vi "LV_vs_PY_timing.vi"() -> ()   [LabVIEW 2021]
panel:
  in  "Fiducials array":path=path "C:/Users/sindh/Desktop/LabVIEW with Python/fiducials.txt"
  out "LV time":dbl
  out "Gantry Fiducials":dbl[](array[numeric])=[574.866049, -722.708823, -78.709075, 574.794272, -905.497716, -78.957629, 575.365932, -722.708925, -78.709081, 575.294318, -905.497893, -78.957622]
  out "XYZTheta":dbl[](array[numeric])
  out "PY time":dbl
  out "XYZTheta 2":dbl[](array[numeric])
  in  "Run LV":bool
  in  "Python version":string="3.6"
  in  "python function name":string="find_component_center"
  in  "python module path":path=path "C:/Users/sindh/Desktop/LabVIEW with Python/test_python.py"
  in  "Run PY":bool
  out "error out":errorcluster
  in  "error in (no error)":errorcluster
  in  "stop":bool
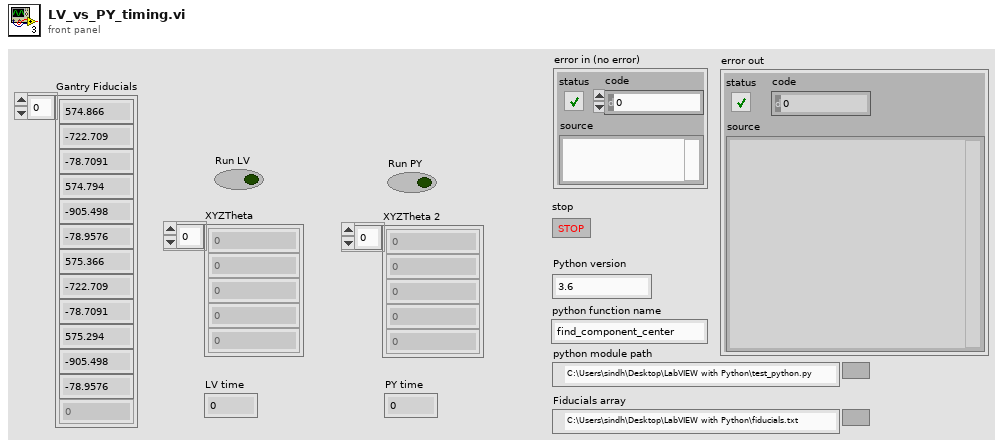
[diagram p1: front panel]
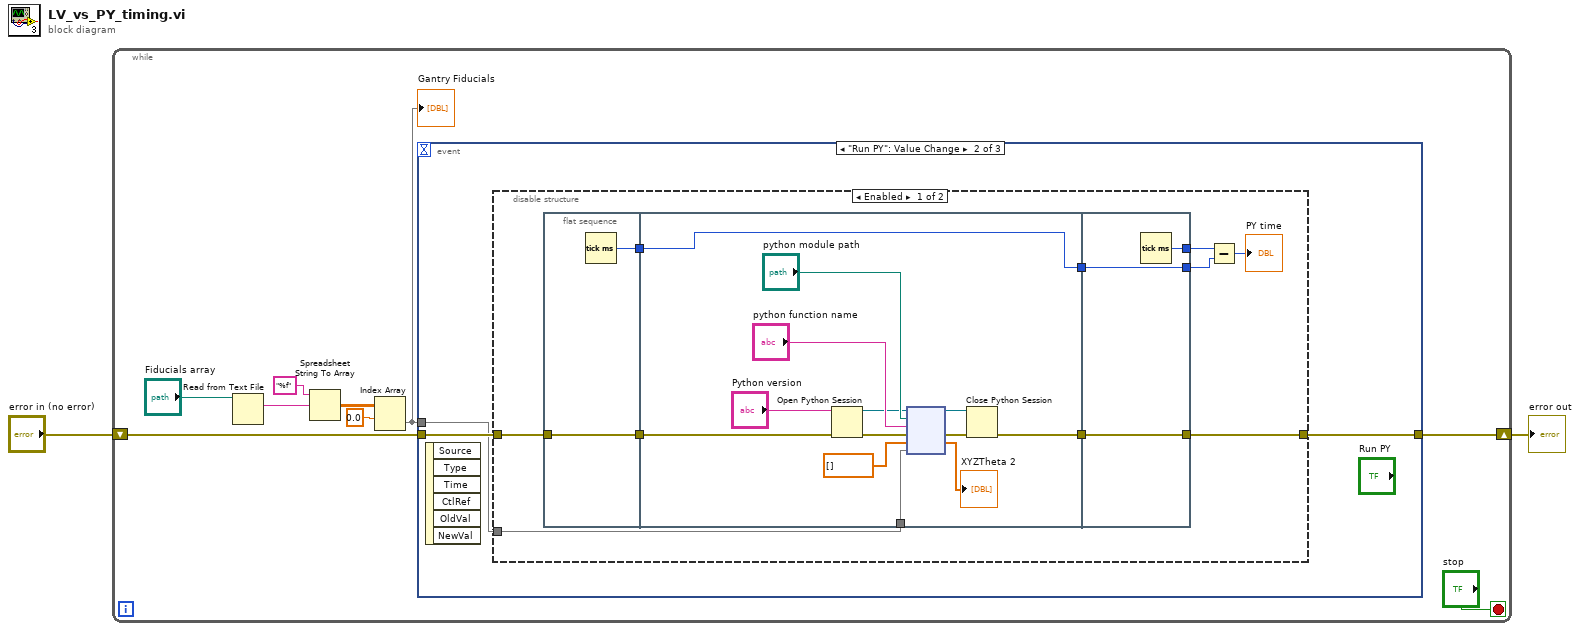
[diagram p0: block diagram]
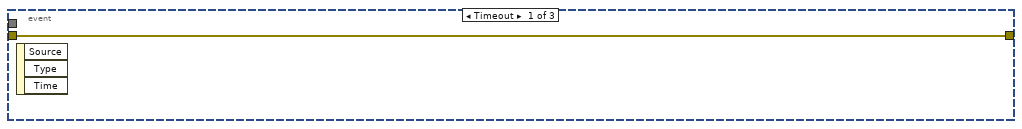
[diagram p2: hidden frame]
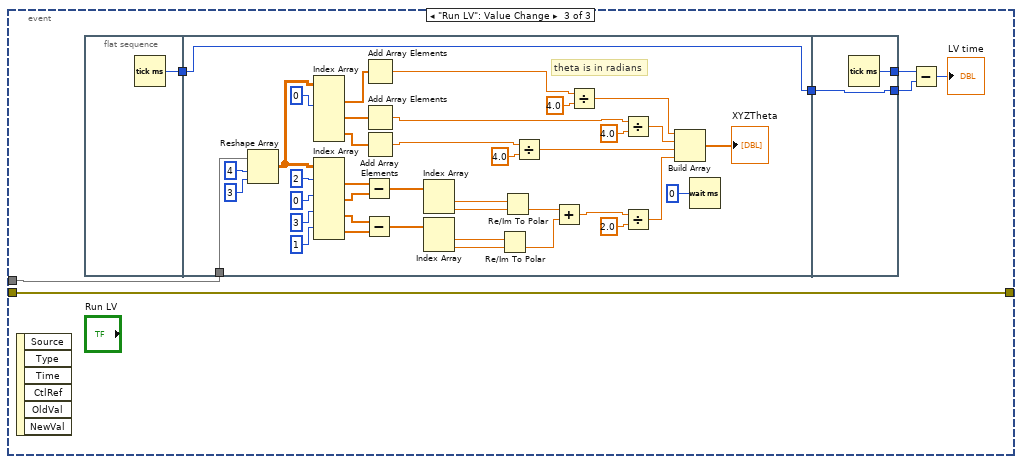
[diagram p4: hidden frame]
diagram:
  n1 = while {
    shift-right: [w10] -> w2
    shift-left: "error in (no error)" -> [w9]
    stop <- "stop" stop-if-true
    n2 = Read from Text File(file (use dialog)="Fiducials array") -> (text=w8:string)  [unwired: 3 in, 3 out]
    n3 = Spreadsheet String To Array(format string="%f", spreadsheet string=w8) -> (array=w5:dbl[][])  [unwired: 2 in]
    n4 = Index Array(array=w5, index (row)=0.0) -> (element=w6:dbl[])  [unwired: 1 in]
    "Gantry Fiducials" <- w6
    n5 = event shown="[1] \"Run PY\": Value Change" {
      selector: _ -> [_ _ _]
      dyn-events: _ -> [_ _ _]
      timeout: _ -> [_ _ _]
      tunnel: w9 -> [w12 w15 w45]
      tunnel: [w12 w14 w45] -> w10
      tunnel: w6 -> [_ w13 w44]
      event Timeout {
        n6 = event-data() -> ()  [unwired: 1 in, 3 out]
      }
      event "Run PY": Value Change {
        n7 = event-data() -> ()  [unwired: 1 in, 6 out]
        n8 = disable-structure shown="Enabled" {
          disable-tunnel: w15 -> [w21 _]
          disable-tunnel: [w20 _] -> w14
          disable-tunnel: w13 -> [w16 _]
          frame Enabled {
            n9 = flat-sequence {
              tunnel: w21 -> [w27]
              tunnel: [w27] -> w25
              tunnel: [w26] -> w24
              tunnel: w25 -> [w35]
              tunnel: [w32] -> w23
              tunnel: [w31] -> w22
              tunnel: w24 -> [w31]
              tunnel: w16 -> [w29]
              tunnel: [w43] -> w20
              tunnel: w23 -> [w43]
              tunnel: [w42] -> w19
              tunnel: [w41] -> w18
              tunnel: w22 -> [w41]
              frame #0 {
                n10 = Tick Count (ms)() -> (millisecond timer value=w26:u32)
              }
              frame #1 {
                n11 = Open Python Session(python version="Python version", 3:w35) -> (session out=w37:refnum<k35>, error out=w34:errorcluster)  [unwired: 1 in]
                n12 = node(w37, "python module path", "python function name", w34, dbl[] [] ("b"), w29) -> (w38:refnum<k35>, w33:errorcluster, →"XYZTheta 2":dbl[])  [unwired: 1 in, 2 out]
                n13 = Close Python Session(session in=w38, error in=w33) -> (11:w32:errorcluster)
              }
              frame #2 {
                n14 = Tick Count (ms)() -> (millisecond timer value=w42:u32)
              }
            }
            n15 = Subtract(x=w19, y=w18) -> (x-y=→"PY time":u32)
          }
          frame Disabled {
          }
        }
      }
      event "Run LV": Value Change {
        n16 = event-data() -> ()  [unwired: 1 in, 6 out]
        n17 = flat-sequence {
          tunnel: [w51] -> w50
          tunnel: [w62] -> w49
          tunnel: w50 -> [w62]
          tunnel: w44 -> [w59]
          tunnel: [w92] -> w48
          tunnel: [w91] -> w47
          tunnel: w49 -> [w91]
          frame #0 {
            n18 = Tick Count (ms)() -> (millisecond timer value=w51:u32)
          }
          frame #1 {
            # "theta is in radians"
            n19 = Reshape Array(w59, 4 ("dimension size"), 3 ("dimension size")) -> (w54:dbl[][])
            n20 = Index Array(array=w54, index (col) #1=0 ("disabled index (col)")) -> (element #1=w57:dbl[], element #2=w89:dbl[], element #3=w64:dbl[])  [unwired: 5 in]
            n21 = Index Array(array=w54, index (row) #1=2 ("index (row)"), index (row) #2=0 ("index (row)"), index (row) #3=3 ("index (row)"), index (row) #4=1 ("index (row)")) -> (element #1=w56:dbl[], element #2=w77:dbl[], element #3=w76:dbl[], element #4=w75:dbl[])  [unwired: 4 in]
            n22 = Subtract(x=w56, y=w77) -> (x-y=w53:dbl[])
            n23 = Subtract(x=w76, y=w75) -> (x-y=w55:dbl[])
            n24 = Add Array Elements(numeric array=w57) -> (sum=w88:dbl)
            n25 = Add Array Elements(numeric array=w89) -> (sum=w87:dbl)
            n26 = Add Array Elements(numeric array=w64) -> (sum=w69:dbl)
            n27 = Index Array(array=w53) -> (element #1=w84:dbl, element #2=w83:dbl)  [unwired: 2 in]
            n28 = Index Array(array=w55) -> (element #1=w82:dbl, element #2=w81:dbl)  [unwired: 2 in]
            n29 = Re/Im To Polar(2:w81, 3:w82) -> (0:w80:dbl)  [unwired: 1 out]
            n30 = Re/Im To Polar(2:w83, 3:w84) -> (0:w52:dbl)  [unwired: 1 out]
            n31 = Divide(x=w69, y=4.0) -> (x/y=w66:dbl)
            n32 = Add(x=w52, y=w80) -> (x+y=w79:dbl)
            n33 = Divide(x=w88, y=4.0) -> (x/y=w68:dbl)
            n34 = Divide(x=w87, y=4.0) -> (x/y=w67:dbl)
            n35 = Divide(x=w79, y=2.0) -> (x/y=w63:dbl)
            n36 = Build Array(w68, w67, w66, w63) -> (→"XYZTheta":dbl[])
            n37 = Wait (ms)(milliseconds to wait=0) -> ()  [unwired: 1 out]
          }
          frame #2 {
            n38 = Tick Count (ms)() -> (millisecond timer value=w92:u32)
          }
        }
        n39 = Subtract(x=w48, y=w47) -> (x-y=→"LV time":u32)
      }
    }
  }
  "error out" <- w2
